vi "Test_DAC_move_overflow.vi"() -> ()   [LabVIEW 2013]
uses:
  <vilib>/Platform/TimedLoop/XDataNode/wakeup.ctl
  <vilib>/Platform/TimedLoop/XDataNode/XDNodeRunTimeDep.lvlib
  <vilib>/Platform/TimedLoop/XDataNode/nitl_modes.ctl
  <vilib>/Platform/TimedLoop/XDataNode/timing_clust.ctl
  <vilib>/Platform/TimedLoop/XDataNode/XDataNode.xnode
  <vilib>/eio/EIONode/EIONode.xnode
  <vilib>/rvi/eio/common/nirviEmuTemplateMethod_errors.vi
  <vilib>/rvi/DataTransferAndStorage/Container/XNode/niFpgaContainer.xnode
  <vilib>/rvi/FIFO/Fifo_Resource/nirvififoEmulationRead.vi
  <vilib>/rvi/FIFO/Fifo_Resource/nirvififoEmulationWrite.vi
panel:
  in  "Channel":u8
  in  "Panel":u8
  in  "Array":u16[](array[numeric])=[0, 6553, 13107, 19660, 26214, 32768, 39321, 45874, 52428, 58982, 65535, 58982, 52428, 45874, 39321, 32768, 26214, 19660, 13107, 6553]
  in  "Count(Ticks)":u32=120
  out "i":i32
  out "Timed Out?":bool
  in  "stop":bool
  # "here"
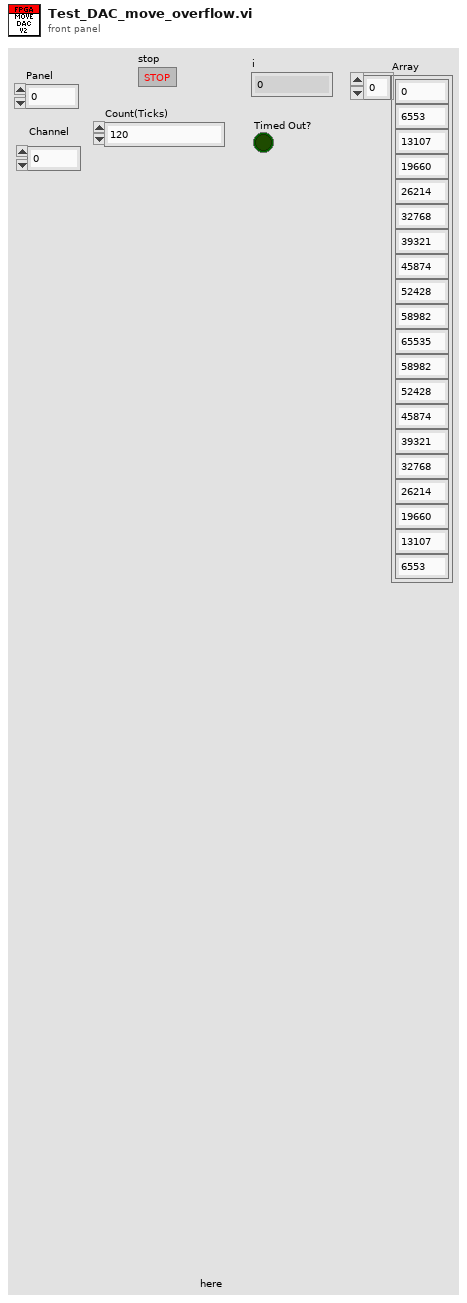
[diagram p1: front panel]
types:
  T1 = typedef "XDNodeRunTimeDep.lvlib/timing_clust.ctl" = cluster{"Expected End [f-1]":u64, "Actual End [f-1]":u64, "Finished Late? [f-1]":bool, "Expected End [i-1]":u64, "Actual End [i-1]":u64, "Finished Late? [i-1]":bool, "Expected Start [i]":u64, "Actual Start [i]":u64, "Expected Start [f]":u64, "Actual Start [f]":u64, "Source Name":string, "Structure Name":string, "Period":i64, "Deadline":i64, "Offset":i64, "Start":i64, "Priority":i32, "Timeout":i32, "Mode":T2, "Wakeup Reason":T3, "Error":errorcluster, "Source Type":string, "Secondary Source Type":string, "Global End Time":u64, "Global Start Time":u64, "Frame Duration":u64, "Iteration Duration":u64, "Assigned CPU":i32, "I/O Scan Engine Mode":u32}
  T2 = typedef "XDNodeRunTimeDep.lvlib/nitl_modes.ctl" = enum32{"No Change", "Process missed periods, maintain original phase", "Discard missed periods, maintain original phase", "Process missed periods, ignore original phase", "Discard missed periods, ignore original phase"}
  T3 = typedef "XDNodeRunTimeDep.lvlib/wakeup.ctl" = enum32{"Normal", "Aborted", "Asynchronous wakeup", "Timing source error", "Timed loop error", "Timeout"}
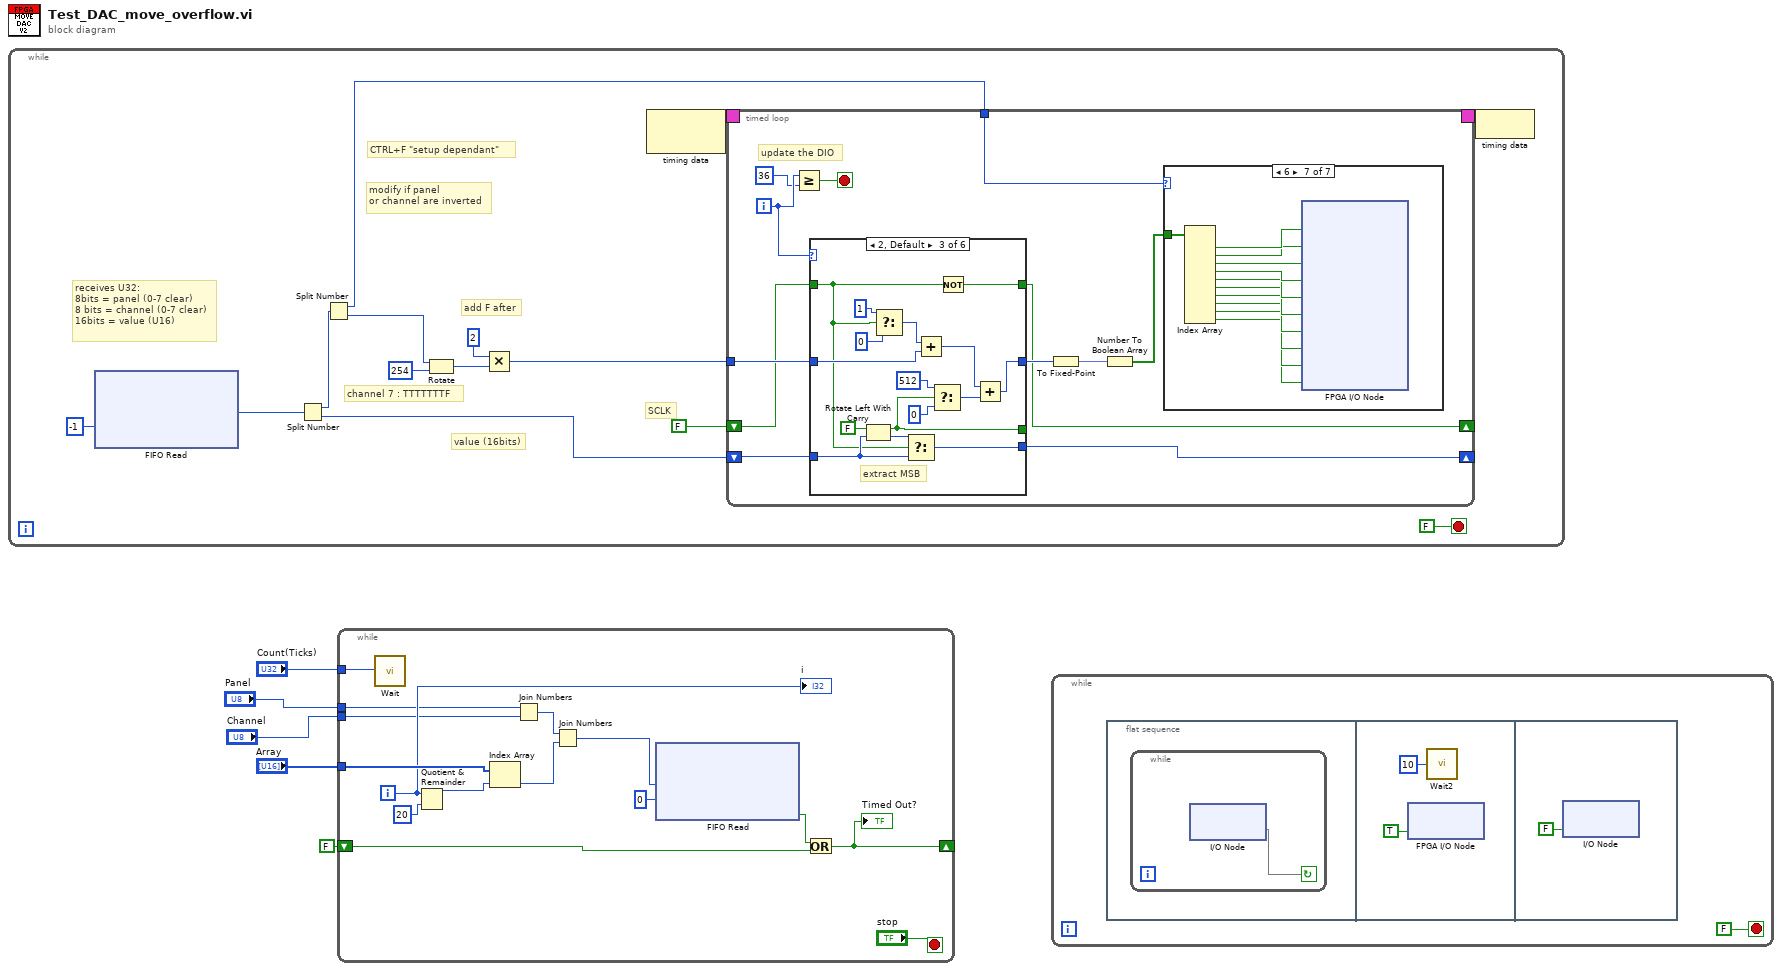
[diagram p0: block diagram]
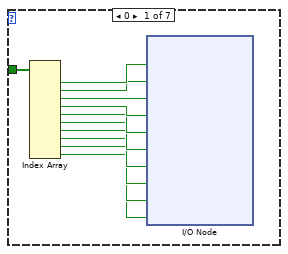
[diagram p2: hidden frame]
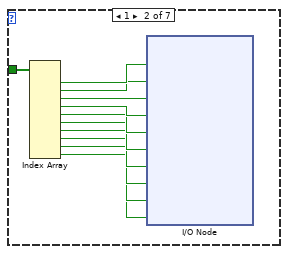
[diagram p3: hidden frame]
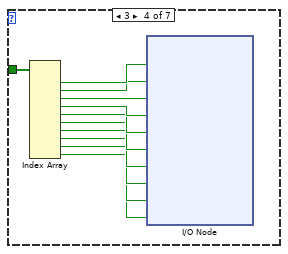
[diagram p5: hidden frame]
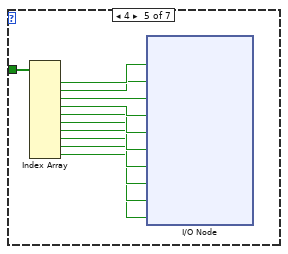
[diagram p6: hidden frame]
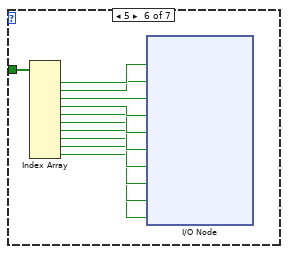
[diagram p7: hidden frame]
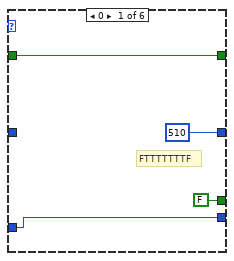
[diagram p8: hidden frame]
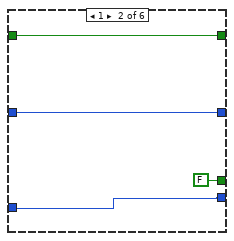
[diagram p9: hidden frame]
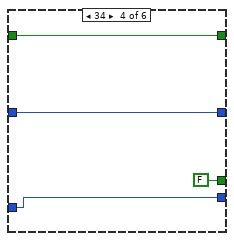
[diagram p10: hidden frame]
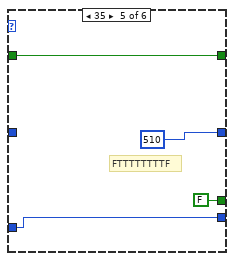
[diagram p11: hidden frame]
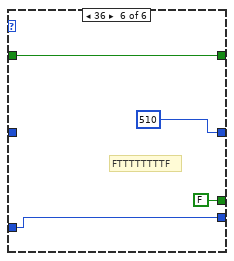
[diagram p12: hidden frame]
diagram:
  n1 = while {
    stop <- FALSE stop-if-true
    # "SCLK"
    # "value (16bits)"
    # "add F after"
    # "channel 7 : TTTTTTTF"
    # "modify if panel\nor channel are inverted"
    # "receives U32:\n8bits = panel (0-7 clear)\n8 bits = channel (0-7 clear)\n16bits = value (U16)"
    # "CTRL+F \"setup dependant\""
    n2 = xnode ("FIFO Read")("Timeout"=-1) -> ("Element"=w19:u32)  [unwired: 1 in, 2 out]
    n3 = Split Number(x=w19) -> (hi(x)=w18:u16, lo(x)=w17:u16)
    n4 = Split Number(x=w18) -> (hi(x)=w9:u8, lo(x)=w8:u8)
    n5 = Rotate(1:u8 254 ("x"), 2:w8) -> (0:w13:u8)
    n6 = Multiply(x=u16 2 ("y"), y=w13) -> (x*y=w16:u16)
    n7 = node-c288() -> (w11:T1)  [unwired: 1 in]
    n8 = timed-loop {
      tunnel: w16 -> [w30]
      shift-right: [w20] -> _
      shift-left: FALSE -> [w29]
      shift-right: [w28] -> _
      shift-left: w17 -> [w31]
      timing: w11 -> [_]
      timing-out: [_] -> w10
      tunnel: w9 -> [w27]
      i -> [w25]
      stop <- w26 stop-if-true
      # "update the DIO"
      n9 = Greater Or Equal?(x=w25, y=36) -> (x >= y?=w26:bool)
      n10 = case shown="2, Default" w25 {
        tunnel: [w101 w105 w121 w125 w129 w133] -> w20
        tunnel: w31 -> [w100 w104 w120 w124 w128 w132]
        tunnel: w30 -> [_ w103 w115 w123 _ _]
        tunnel: w29 -> [w101 w105 w113 w125 w129 w133]
        tunnel: [w100 w104 w112 w124 w128 w132] -> w28
        tunnel: [u16 510 w103 w107 w123 u16 510 ("t") u16 510 ("t")] -> w22
        tunnel: [FALSE ("msb carry out") FALSE ("msb carry out") w106 FALSE ("msb carry out") FALSE ("msb carry out") FALSE ("msb carry out")] -> _
        frame 0 {
          # "FTTTTTTTF"
        }
        frame 1 {
        }
        frame 2, Default {
          # "extract MSB"
          n11 = Rotate Left With Carry(2:w120, 3:FALSE ("carry")) -> (0:w119:u16, 1:w106:bool)
          n12 = Select(t=u16 1, s=w113, f=u16 0 ("t")) -> (s? t:f=w116:u16)
          n13 = Select(t=w119, s=w113, f=w120) -> (s? t:f=w112:u16)
          n14 = Add(x=w116, y=w115) -> (x+y=w111:u16)
          n15 = Select(t=u16 512, s=w106, f=u16 0 ("t")) -> (s? t:f=w110:u16)
          n16 = Not(x=w113) -> (.not. x?=w121:bool)
          n17 = Add(x=w111, y=w110) -> (x+y=w107:u16)
        }
        frame 34 {
        }
        frame 35 {
          # "FTTTTTTTTF"
        }
        frame 36 {
          # "FTTTTTTTTF"
        }
      }
      n18 = To Fixed-Point(number=w22) -> (fixed-point=w21:fxp<+,10,10>)  [unwired: 1 in]
      n19 = Number To Boolean Array(number=w21) -> (Boolean array=w23:bool[])
      n20 = case shown="6" w27 {
        tunnel: w23 -> [w42 w53 _ w64 w75 w86 w97]
        frame 0 {
          n21 = Index Array(array=w42) -> (element #1=w41:bool, element #2=w40:bool, element #3=w39:bool, element #4=w38:bool, element #5=w37:bool, element #6=w36:bool, element #7=w35:bool, element #8=w34:bool, element #9=w33:bool, element #10=w32:bool)  [unwired: 10 in]
          n22 = xnode "I/O Node"("RMC/DIO12"=w41, "RMC/DIO76"=w40, "RMC/DIO44"=w39, "RMC/DIO13"=w38, "RMC/DIO45"=w37, "RMC/DIO14"=w36, "RMC/DIO46"=w35, "RMC/DIO77"=w34, "RMC/DIO15"=w33, "RMC/DIO43"=w32) -> ()  [unwired: 10 in, 10 out]
        }
        frame 1 {
          n23 = Index Array(array=w53) -> (element #1=w52:bool, element #2=w51:bool, element #3=w50:bool, element #4=w49:bool, element #5=w48:bool, element #6=w47:bool, element #7=w46:bool, element #8=w45:bool, element #9=w44:bool, element #10=w43:bool)  [unwired: 10 in]
          n24 = xnode "I/O Node"("RMC/DIO8"=w52, "RMC/DIO72"=w51, "RMC/DIO40"=w50, "RMC/DIO9"=w49, "RMC/DIO41"=w48, "RMC/DIO10"=w47, "RMC/DIO74"=w46, "RMC/DIO42"=w45, "RMC/DIO11"=w44, "RMC/DIO39"=w43) -> ()  [unwired: 10 in, 10 out]
        }
        frame 2, Default {
          # "2, 7, 8 and 9 are not connected"
        }
        frame 3 {
          n25 = Index Array(array=w64) -> (element #1=w63:bool, element #2=w62:bool, element #3=w61:bool, element #4=w60:bool, element #5=w59:bool, element #6=w58:bool, element #7=w57:bool, element #8=w56:bool, element #9=w55:bool, element #10=w54:bool)  [unwired: 10 in]
          n26 = xnode "I/O Node"("RMC/DIO4"=w63, "RMC/DIO69"=w62, "RMC/DIO36"=w61, "RMC/DIO5"=w60, "RMC/DIO37"=w59, "RMC/DIO6"=w58, "RMC/DIO70"=w57, "RMC/DIO38"=w56, "RMC/DIO7"=w55, "RMC/DIO35"=w54) -> ()  [unwired: 10 in, 10 out]
        }
        frame 4 {
          n27 = Index Array(array=w75) -> (element #1=w74:bool, element #2=w73:bool, element #3=w72:bool, element #4=w71:bool, element #5=w70:bool, element #6=w69:bool, element #7=w68:bool, element #8=w67:bool, element #9=w66:bool, element #10=w65:bool)  [unwired: 10 in]
          n28 = xnode "I/O Node"("RMC/DIO66"=w74, "RMC/DIO65"=w73, "RMC/DIO32"=w72, "RMC/DIO33"=w71, "RMC/DIO1"=w70, "RMC/DIO67"=w69, "RMC/DIO34"=w68, "RMC/DIO68"=w67, "RMC/DIO3"=w66, "RMC/DIO64"=w65) -> ()  [unwired: 10 in, 10 out]
        }
        frame 5 {
          n29 = Index Array(array=w86) -> (element #1=w85:bool, element #2=w84:bool, element #3=w83:bool, element #4=w82:bool, element #5=w81:bool, element #6=w80:bool, element #7=w79:bool, element #8=w78:bool, element #9=w77:bool, element #10=w76:bool)  [unwired: 10 in]
          n30 = xnode "I/O Node"("RMC/DIO26"=w85, "RMC/DIO91"=w84, "RMC/DIO58"=w83, "RMC/DIO57"=w82, "RMC/DIO90"=w81, "RMC/DIO25"=w80, "RMC/DIO89"=w79, "RMC/DIO56"=w78, "RMC/DIO55"=w77, "RMC/DIO92"=w76) -> ()  [unwired: 10 in, 10 out]
        }
        frame 6 {
          n31 = Index Array(array=w97) -> (element #1=w96:bool, element #2=w95:bool, element #3=w94:bool, element #4=w93:bool, element #5=w92:bool, element #6=w91:bool, element #7=w90:bool, element #8=w89:bool, element #9=w88:bool, element #10=w87:bool)  [unwired: 10 in]
          n32 = xnode "FPGA I/O Node"("RMC/DIO30"=w96, "RMC/DIO95"=w95, "RMC/DIO29"=w94, "RMC/DIO28"=w93, "RMC/DIO94"=w92, "RMC/DIO60"=w91, "RMC/DIO93"=w90, "RMC/DIO59"=w89, "RMC/DIO27"=w88, "RMC/DIO31"=w87) -> ()  [unwired: 10 in, 10 out]
        }
      }
    }
    n33 = node-c288(w10) -> ()
  }
  n34 = while {
    shift-right: [w145] -> _
    shift-left: FALSE -> [w146]
    tunnel: "Count(Ticks)" -> [w144]
    tunnel: "Array" -> [w142]
    tunnel: "Channel" -> [w139]
    tunnel: "Panel" -> [w138]
    i -> [w140]
    stop <- "stop" stop-if-true
    n35 = call "Wait"("Count(Ticks)"=w144) -> ()  [unwired: 1 out]
    n36 = Quotient & Remainder(x=w140, y=20) -> (x-y*floor(x/y)=w143:i32)  [unwired: 1 out]
    n37 = Index Array(array=w142, index=w143) -> (element=w141:u16)
    n38 = Join Numbers(hi=w138, lo=w139) -> ((hi.lo)=w152:u16)
    n39 = Join Numbers(hi=w152, lo=w141) -> ((hi.lo)=w151:u32)
    n40 = xnode ("FIFO Read")("Element"=w151, "Timeout"=0) -> ("Timed Out?"=w147:bool)  [unwired: 1 in, 1 out]
    n41 = Or(x=w147, y=w146) -> (x .or. y?=w145:bool)
    "Timed Out?" <- w145
    "i" <- w140
  }
  n42 = while {
    stop <- FALSE stop-if-true
    n43 = flat-sequence {
      frame #0 {
        n44 = while {
          stop <- w154 continue-if-true
          n45 = xnode "I/O Node"() -> ("DIO2"=w154)  [unwired: 1 in, 1 out]
        }
      }
      frame #1 {
        n46 = xnode "FPGA I/O Node"("DIO0"=TRUE) -> ()  [unwired: 1 in, 1 out]
        n47 = call "Wait2"("Count(uSec)"=u32 10) -> ()  [unwired: 1 out]
      }
      frame #2 {
        n48 = xnode "I/O Node"("DIO0"=FALSE) -> ()  [unwired: 1 in, 1 out]
      }
    }
  }
